vi "sqlDriver.vi"(6 "SQL Driver Selection Driver":T1, 8 "Error In":errorcluster, 10 "Query":string, 11 "Database File Path":path) -> (0 "Error Out":errorcluster, 3 "Result Table":string[][](array[string]))   [LabVIEW 2018]
uses:
  controls/sqlDriverSelectionEnum.ctl
  <vilib>/addons/database/Connection.llb/DB Tools Open Connec (Path).vi
  <vilib>/addons/database/Connection.llb/Conn Execute.vi
  <vilib>/addons/database/Recordset.llb/Rec Fetch Recordset Data (R).vi
  <vilib>/addons/database/Recordset.llb/Rec Destroy - Connection.vi
  <vilib>/addons/database/_DB Variant To Data/Database Variant To Data.xnode
  <vilib>/addons/database/NI_Database_API.lvlib
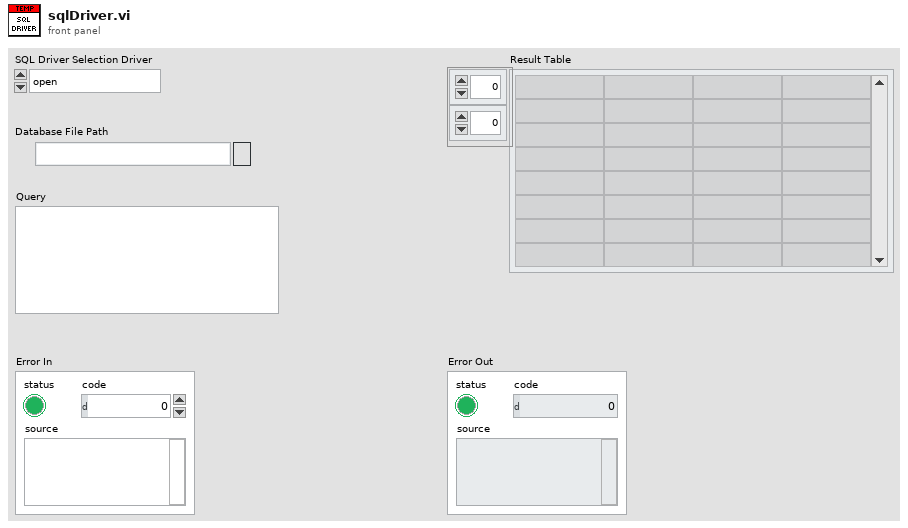
[diagram p1: front panel]
types:
  T1 = typedef "sqlDriverSelectionEnum.ctl" = enum16{"open", "query & fetch", "close"}
  T2 = typedef "NI_Database_API.lvlib/Conn ObjectReference.ctl" = refnum<k1>
  T3 = typedef "NI_Database_API.lvlib/Rec ObjectReference.ctl" = refnum<k1>
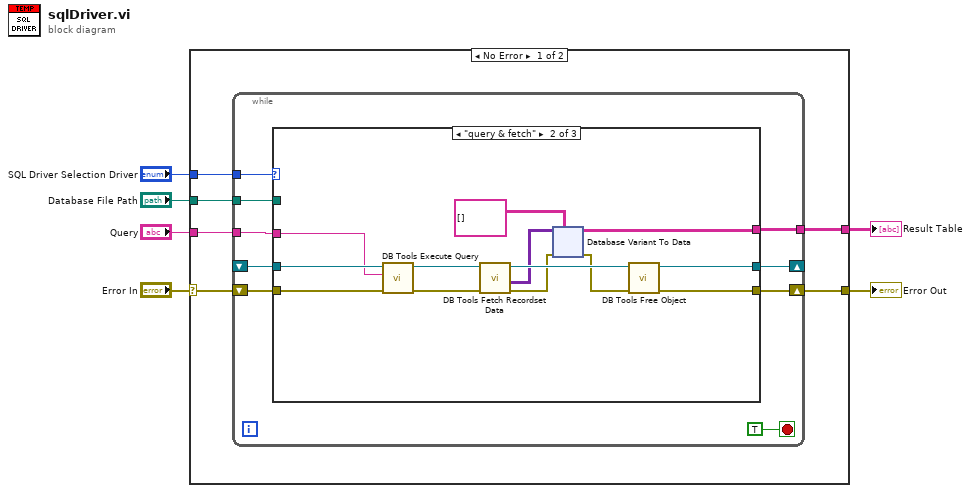
[diagram p0: block diagram]
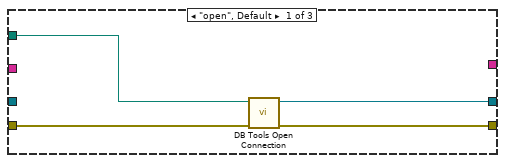
[diagram p2: hidden frame]
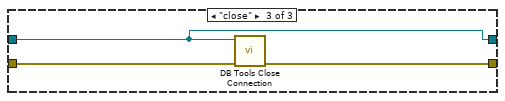
[diagram p3: hidden frame]
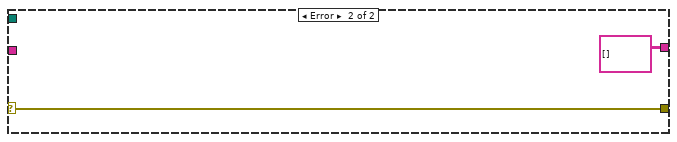
[diagram p4: hidden frame]
diagram:
  n1 = case shown="No Error" "Error In" {
    selector: "Error In" -> [w12 w87]
    tunnel: [w11 w87] -> w4
    tunnel: [w10 string[][] [] ("data")] -> w1
    tunnel: "Database File Path" -> [w9 _]
    tunnel: "SQL Driver Selection Driver" -> [w8 _]
    tunnel: "Query" -> [w7 _]
    frame No Error {
      n2 = while {
        shift-right: [w20] -> w11
        shift-left: w12 -> [w21]
        shift-right: [w18] -> _
        shift-left: _ -> [w17]
        tunnel: [w16] -> w10
        tunnel: w9 -> [w15]
        tunnel: w8 -> [w14]
        tunnel: w7 -> [w13]
        stop <- TRUE stop-if-true
        n3 = case shown="\"query & fetch\"" w14 {
          tunnel: w21 -> [w24 w38 w84]
          tunnel: [w25 w35 w85] -> w20
          tunnel: [w23 w36 w83] -> w18
          tunnel: w17 -> [_ w37 w83]
          tunnel: [_ w27 _] -> w16
          tunnel: w15 -> [w22 _ _]
          tunnel: w13 -> [_ w26 _]
          frame "open", Default {
            n4 = call-poly <vilib>:"DB Tools Open Connection.vi"("error in (no error)"=w24, "connection information"=w22) -> ("error out"=w25:errorcluster, "connection reference"=w23:T2)  [unwired: 6 in]
          }
          frame "query & fetch" {
            n5 = call-poly <vilib>:"DB Tools Execute Query.vi"("error in (no error)"=w38, "SQL query"=w26, "connection reference"=w37) -> ("error out"=w34:errorcluster, "recordset reference"=w33:T3)  [unwired: 5 in]
            n6 = call-poly <vilib>:"DB Tools Fetch Recordset Data.vi"("error in (no error)"=w34, "recordset reference"=w33) -> ("error out"=w30:errorcluster, "recordset data"=w31:variant[][], "recordset reference out"=w32:T3)  [unwired: 3 in]
            n7 = xnode "Database Variant To Data"("database variant"=w31, "error in (no error)"=w30, "type"=string[][] []) -> ("data"=w27:string[][], "error out"=w29:errorcluster)
            n8 = call-poly <vilib>:"DB Tools Free Object.vi"("error in (no error)"=w29, "recordset reference"=w32) -> ("error out"=w35:errorcluster, "connection reference"=w36:T2)  [unwired: 8 in]
          }
          frame "close" {
            n9 = call <vilib>:"DB Tools Close Connection.vi"("error in (no error)"=w84, "connection reference"=w83) -> ("error out"=w85:errorcluster)  [unwired: 5 in]
          }
        }
      }
    }
    frame Error {
    }
  }
  "Error Out" <- w4
  "Result Table" <- w1
